vi "Yokogawa - Settingsvi.vi"(8 "error in (no error)":errorcluster, 11 "Hardware Configuration":T1={"VISA resource name"="", "Mode (0: Normal) "=0, "Voltage"={"Element (0: All)"=0, "V Range (200)"=4}, "Current"={"A Range (2)"=7, "A Terminal (0: 5A)"=0, "Element (0: ALL)"=0}, "Observation Time"=10, "Modules on/off"={"Module 1"=FALSE, "Module 2"=FALSE, "Module 3"=FALSE, "Module 4"=FALSE}} {"Observation Time" items=["1ksec", "400sec", "200sec", "100sec", "40sec", "20sec", "10sec", "4sec", "2sec", "1sec", "400msec", "200msec", "100msec", "40msec", "20msec", "10msec", "4msec", "2msec", "1msec", "400usec", "200usec", "100usec", "40usec", "20usec", "10usec"]; "Mode (0: Normal)" items=["Normal", "Harmonics"]; "Current"."Element (0: ALL)" items=["All", "Element 1", "Element 2", "Element 3", "Element 4"]; "Current"."A Terminal (0: 5A)" items=["5A", "20A", "Sensor"]; "Current"."A Range (2)" items=["AUTO", "0.1", "0.2", "0.4", "1", "2", "4", "10", "20", "40", "100"]; "Voltage"."V Range (200)" items=["AUTO", "30", "60", "120", "200", "300", "600", "1200", "2000"]; "Voltage"."Element (0: All)" items=["All", "Element 1", "Element 2", "Element 3", "Element 4"]}) -> (0 "error out 2":errorcluster, 3 "VISA resource name out":refnum<visa-resource-name>)   [LabVIEW 2013]
uses:
  Acquisition/Hardware Configuration.ctl
  <instrlib>/Yokogawa PZ4000/Yokogawa PZ4000.lvlib
  Acquisition/YKPZ400 Acquisition.lvlib
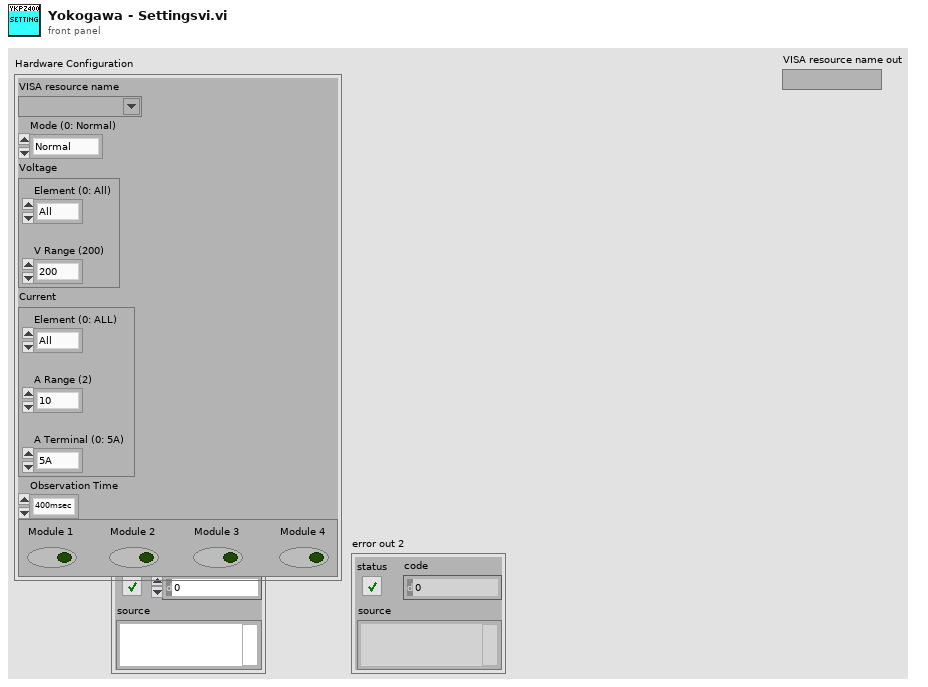
[diagram p1: front panel]
types:
  T1 = typedef "YKPZ400 Acquisition.lvlib/Hardware Configuration.ctl" = cluster{"VISA resource name":refnum<visa-resource-name>, "Mode (0: Normal) ":u16, "Voltage":cluster{"Element (0: All)":u16, "V Range (200)":u16}, "Current":cluster{"A Range (2)":u16, "A Terminal (0: 5A)":u16, "Element (0: ALL)":u16}, "Observation Time":u16, "Modules on/off":cluster{"Module 1":bool, "Module 2":bool, "Module 3":bool, "Module 4":bool}}
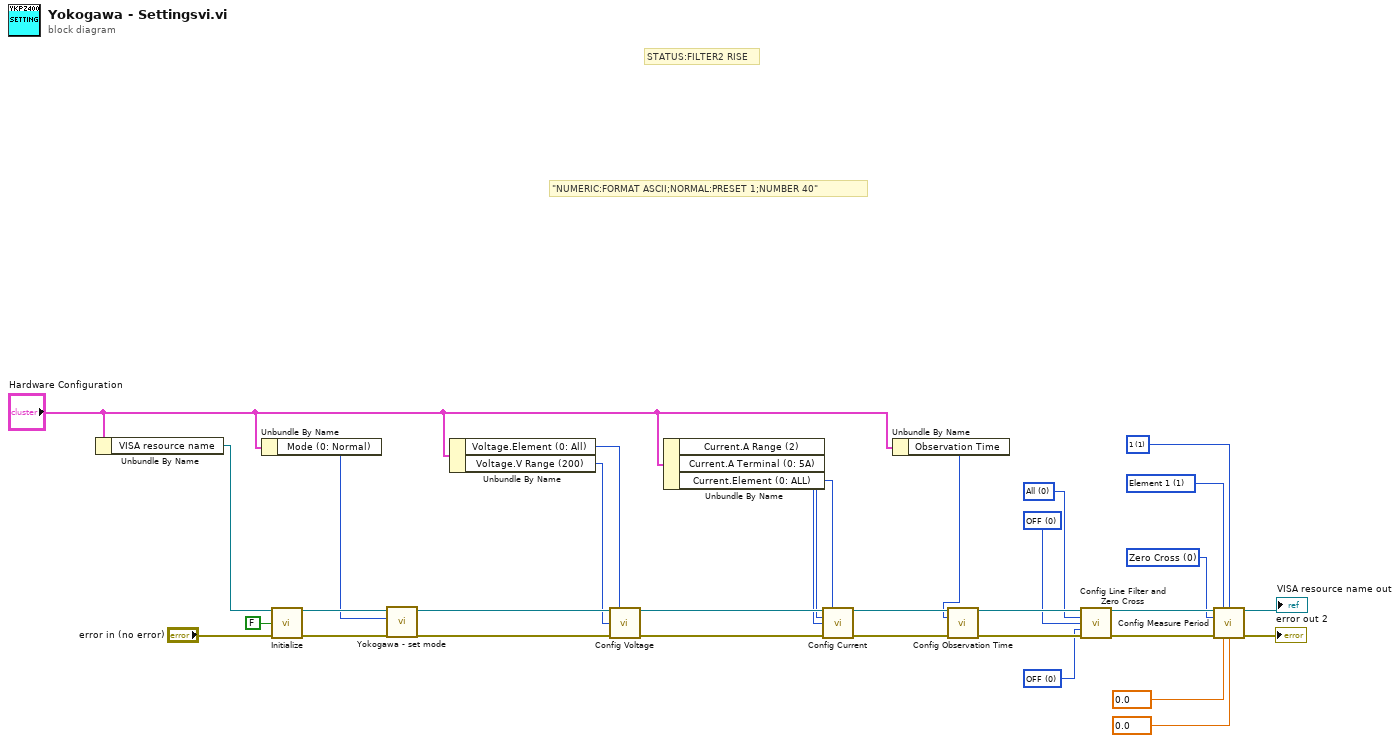
[diagram p0: block diagram]
diagram:
  w13 = u16 0 items=["Zero Cross", "Cursor", "Ext Trigger"] ("Period Mode (0: Zero Cross)")
  w16 = u16 1 items=["", "Element 1", "Element 2", "Element 3", "Element 4"] ("Element (1: Element 1)")
  w12 = u16 1 items=["", "1", "2", "3", "4", "5", "6", "7", "8", "Ext"] ("Synchronize Source (1: 1)")
  w21 = u16 0 items=["All", "Element 1", "Element 2", "Element 3", "Element 4"] ("Element (0: ALL) 2")
  w20 = u16 0 items=["OFF", "500Hz", "20kHz", "1MHz"] ("Line Filter (0: OFF)")
  w19 = u16 0 items=["OFF", "500Hz", "20kHz"] ("Zero Cross Filter (0: OFF)")
  # "\"NUMERIC:FORMAT ASCII;NORMAL:PRESET 1;NUMBER 40\""
  # "STATUS:FILTER2 RISE"
  n1 = Unbundle By Name("Hardware Configuration") -> ("VISA resource name"=w1:refnum<visa-resource-name>)
  n2 = Unbundle By Name("Hardware Configuration") -> ("Mode (0: Normal)"=w9:u16)
  n3 = call <instrlib>:"Initialize.vi"("VISA resource name"=w1, "Reset (T: Reset)"=FALSE, "error in (no error)"="error in (no error)") -> ("VISA resource name out"=w30:refnum<visa-resource-name>, "error out"=w29:errorcluster)  [unwired: 11 in]
  n4 = call "Yokogawa - set mode.vi"("error in (no error)"=w29, "Mode (0: Normal)"=w9, "VISA Refnum in"=w30) -> ("error out"=w10:errorcluster, "VISA Refnum out"=w11:refnum<visa-resource-name>)  [unwired: 7 in]
  n5 = Unbundle By Name("Hardware Configuration") -> ("Voltage.Element (0: All)"=w5:u16, "Voltage.V Range (200)"=w4:u16)
  n6 = call <instrlib>:"Config Voltage.vi"("VISA resource name"=w11, "Element (0: All)"=w5, "V Range (8: 2000)"=w4, "error in (no error)"=w10) -> ("VISA resource name out"=w32:refnum<visa-resource-name>, "error out"=w31:errorcluster)  [unwired: 10 in]
  n7 = Unbundle By Name("Hardware Configuration") -> ("Current.A Range (2)"=w6:u16, "Current.A Terminal (0: 5A)"=w7:u16, "Current.Element (0: ALL)"=w8:u16)
  n8 = call <instrlib>:"Config Current.vi"("VISA resource name"=w32, "Element (0: ALL)"=w8, "A Terminal (0: 5A)"=w7, "A Range (7:10)"=w6, "error in (no error)"=w31) -> ("VISA resource name out"=w25:refnum<visa-resource-name>, "error out"=w23:errorcluster)  [unwired: 9 in]
  n9 = Unbundle By Name("Hardware Configuration") -> ("Observation Time"=w3:u16)
  n10 = call <instrlib>:"Config Observation Time.vi"("VISA resource name"=w25, "Observation Time (12: 100msec)"=w3, "error in (no error)"=w23) -> ("VISA resource name out"=w24:refnum<visa-resource-name>, "error out"=w22:errorcluster)  [unwired: 11 in]
  n11 = call <instrlib>:"Config Line Filter and Zero Cross.vi"("VISA resource name"=w24, "Element (0: ALL)"=w21, "Line Filter (0: OFF)"=w20, "Zero Cross Filter (0: OFF)"=w19, "error in (no error)"=w22) -> ("VISA resource name out"=w18:refnum<visa-resource-name>, "error out"=w17:errorcluster)  [unwired: 9 in]
  n12 = call <instrlib>:"Config Measure Period.vi"("VISA resource name"=w18, "Element (1: Element 1)"=w16, "Synchronize Source (1: 1)"=w12, "Period Mode (0: Zero Cross)"=w13, "error in (no error)"=w17, "From (0)"=0.0, "To (0)"=0.0) -> ("VISA resource name out"=→"VISA resource name out":refnum<visa-resource-name>, "error out"=→"error out 2":errorcluster)  [unwired: 7 in]
